vi "Cal Aux Corrections.vi"(8 "error in (no error)":errorcluster, 10 "Spectral distribution":cluster{dbl, dbl}[](graph)) -> (0 "error out":errorcluster)   [LabVIEW 2013, in "AvaSpec Acquisition.lvlib"]
uses:
  Acquisition/AvaSpec Acquisition.lvlib
  Acquisition/Hardware Configuration.ctl
  Libraries/AS-5216-DLL/AVS settings.ctl
  Acquisition/Sphere Indicator.ctl
  <vilib>/Utility/file.llb/Read From Spreadsheet File (DBL).vi
  Libraries/IRRAD-DLL/AVSirrad.lvlib
panel:
  out "Spectral distribution 2":cluster{dbl, dbl}[](graph)
  out "Hardware Resources out":T1
  in  "Hardware Resources in":T1
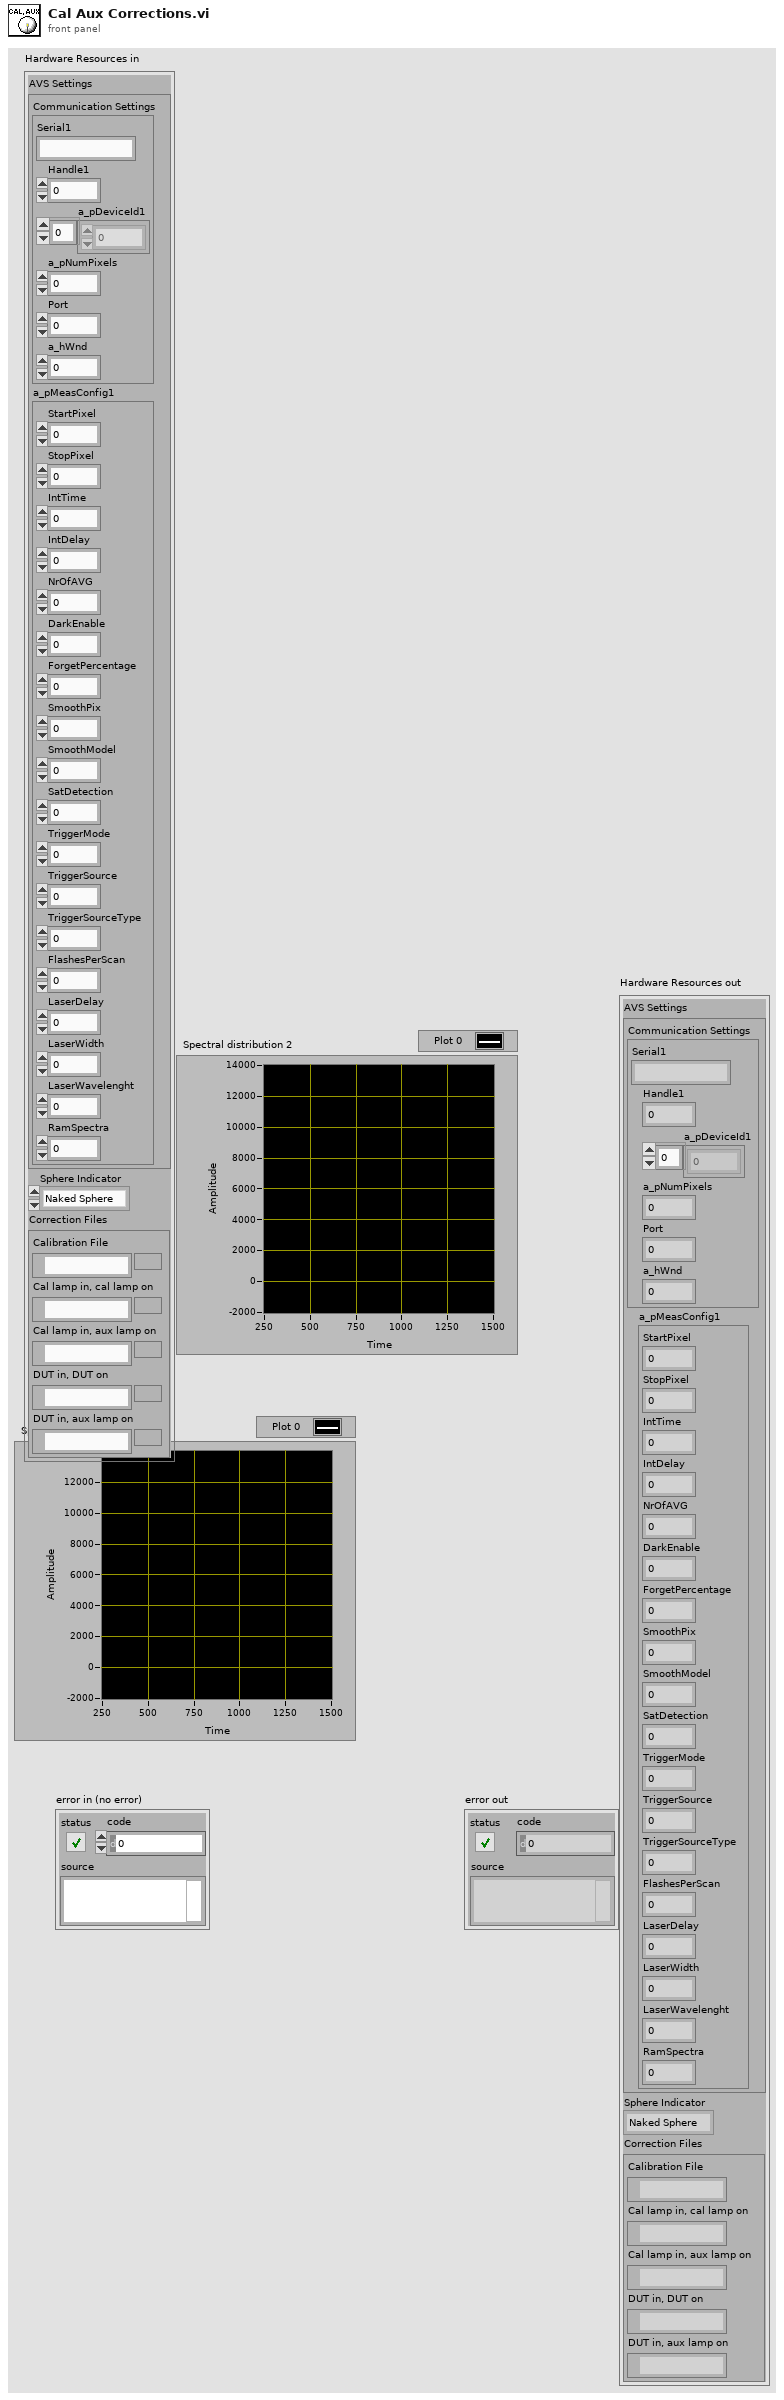
[diagram p1: front panel]
types:
  T1 = typedef "AvaSpec Acquisition.lvlib/Hardware Configuration.ctl" = cluster{"AVS Settings":T2, "Sphere Indicator":T3, "Correction Files":cluster{"Calibration File":path, "Cal lamp in, cal lamp on":path, "Cal lamp in, aux lamp on":path, "DUT in, DUT on":path, "DUT in, aux lamp on":path}}
  T2 = typedef "AVSirrad.lvlib/AVS settings.ctl" = cluster{"Communication Settings":cluster{"Serial1":string, "Handle1":i32, "a_pDeviceId1":u8[], "a_pNumPixels":u16, "Port":i32, "a_hWnd":i32}, "a_pMeasConfig1":cluster{"StartPixel":u16, "StopPixel":u16, "IntTime":sgl, "IntDelay":u32, "NrOfAVG":u32, "DarkEnable":u8, "ForgetPercentage":u8, "SmoothPix":u16, "SmoothModel":u8, "SatDetection":u8, "TriggerMode":u8, "TriggerSource":u8, "TriggerSourceType":u8, "FlashesPerScan":u16, "LaserDelay":u32, "LaserWidth":u32, "LaserWavelenght":sgl, "RamSpectra":u16}}
  T3 = typedef "Sphere Indicator.ctl" = enum16{"Naked Sphere", "Insulated Sphere"}
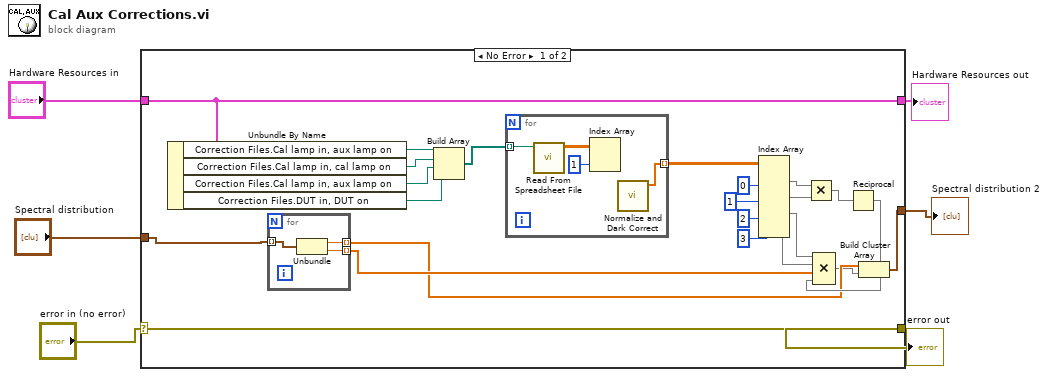
[diagram p0: block diagram]
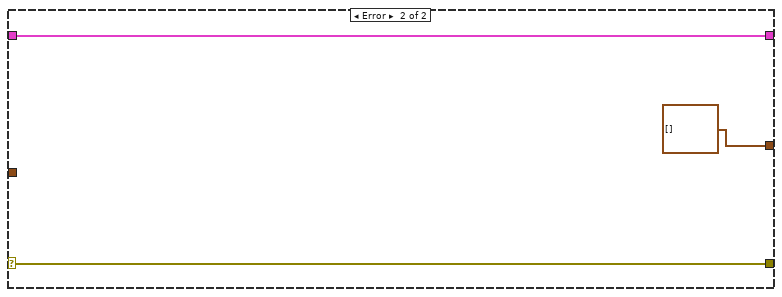
[diagram p2: hidden frame]
diagram:
  n1 = case shown="No Error" "error in (no error)" {
    selector: "error in (no error)" -> [w29 w39]
    tunnel: [w29 w39] -> w5
    tunnel: "Spectral distribution" -> [w22 _]
    tunnel: "Hardware Resources in" -> [w28 w38]
    tunnel: [w28 w38] -> w2
    tunnel: [w7 cluster{dbl, dbl}[] [] ("Spectral distribution 3")] -> w1
    frame No Error {
      n2 = Unbundle By Name(w28) -> ("Correction Files.Cal lamp in, aux lamp on"=w27:path, "Correction Files.Cal lamp in, cal lamp on"=w26:path, "Correction Files.Cal lamp in, aux lamp on"=w25:path, "Correction Files.DUT in, DUT on"=w24:path)
      n3 = for {
        tunnel: w22 -> [w32] mode=indexing
        tunnel: [w31] -> w11 mode=indexing
        tunnel: [w30] -> w9 mode=indexing
        n4 = Unbundle(w32) -> (w30:dbl, w31:dbl)
      }
      n5 = Build Array(w27, w26, w25, w24) -> (w23:path[])
      n6 = for {
        tunnel: w23 -> [w34] mode=indexing
        tunnel: [w33] -> w21 mode=indexing
        n7 = call-poly <vilib>:"Read From Spreadsheet File.vi"("file path (dialog if empty)"=w34) -> ("all rows"=w36:dbl[][])  [unwired: 6 in, 4 out]
        n8 = Index Array(array=w36, index (col)=1 ("disabled index (col)")) -> ()  [unwired: 1 in, 1 out]
        n9 = call "Normalize and Dark Correct.vi"() -> ("Normalized and Dark Corrected"=w33:dbl[])  [unwired: 11 in]
      }
      n10 = Index Array(array=w21, index (col) #1=0 ("disabled index (col)"), index (col) #2=1 ("index (col)"), index (col) #3=2 ("index (col)"), index (col) #4=3 ("index (col)")) -> (element #1=w16:dbl[], element #2=w15:dbl[], element #3=w13:dbl[], element #4=w12:dbl[])  [unwired: 4 in]
      n11 = Multiply(x=w16, y=w15) -> (x*y=w14:dbl[])
      n12 = Reciprocal(x=w14) -> (1/x=w10:dbl[])
      n13 = Compound Arithmetic op=MULTIPLY(w13, w12, w11, w10) -> (w8:dbl[])
      n14 = Build Cluster Array(w9, w8) -> (w7:cluster{dbl, dbl}[])
    }
    frame Error {
    }
  }
  "error out" <- w5
  "Hardware Resources out" <- w2
  "Spectral distribution 2" <- w1
